vi "GetParam.vi"(8 "error in (no error)":errorcluster caption="entrée d'erreur (pas d'erreur)", 11 "MaxAbsScaler.lvclass":refnum<class "MaxAbsScaler.lvclass">) -> (0 "error out":errorcluster caption="sortie d'erreur", 2 "MaxAbsScaler":cluster{"copy":bool}={"copy"=TRUE}, 3 "MaxAbsScaler.lvclass":refnum<class "MaxAbsScaler.lvclass">)   [LabVIEW 2020, in "MaxAbsScaler.lvclass"]
doc: "Get Parameters"
uses:
  MaxAbsScaler.lvclass
  MaxAbsScaler.lvclass/MaxAbsScaler.ctl
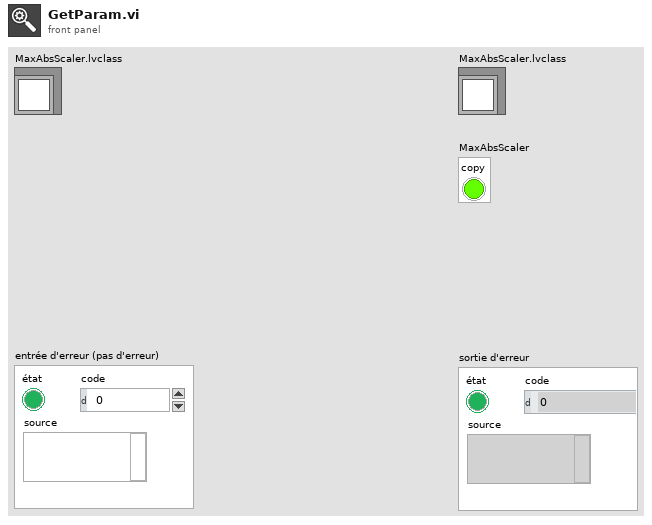
[diagram p1: front panel]
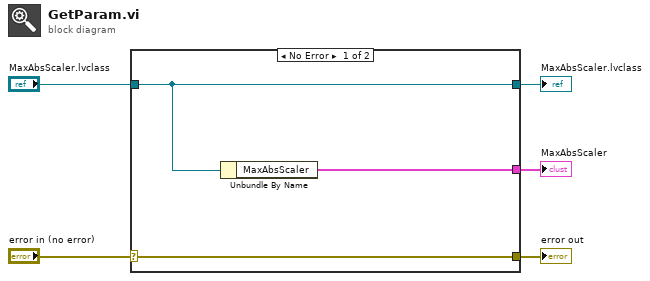
[diagram p0: block diagram]
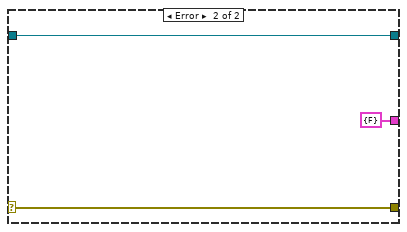
[diagram p2: hidden frame]
diagram:
  n1 = case shown="No Error" "error in (no error)" {
    selector: "error in (no error)" -> [w8 w10]
    tunnel: [w8 w10] -> w4
    tunnel: [w7 w11] -> w2
    tunnel: "MaxAbsScaler.lvclass" -> [w7 w11]
    tunnel: [w6 cluster{"copy":bool} {"copy"=FALSE} ("MaxAbsScaler")] -> w1
    frame No Error {
      n2 = Unbundle By Name(w7) -> ("MaxAbsScaler"=w6:cluster{"copy":bool})
    }
    frame Error {
    }
  }
  "error out" <- w4
  "MaxAbsScaler.lvclass" <- w2
  "MaxAbsScaler" <- w1
